vi "PIM Set Plot Colors.vi"(5 "PEAK IM":refnum<vi>, 7 "IM Plot":refnum<vi>, 8 "IM Order (0)":u8, 9 "IM In Band? (F, F, F, F)":bool[](array[boolean]), 10 "Markers Visible?":bool, 11 "DisplayMode":T1 items=["Spectral", "Strip Chart", "Swept Frequency"]) -> (2 "Mrkr Text Colors":u32[](array[numeric]), 3 "Marker Colors":u32[](array[numeric]))   [LabVIEW 2011]
uses:
  PIM Display Mode.ctl
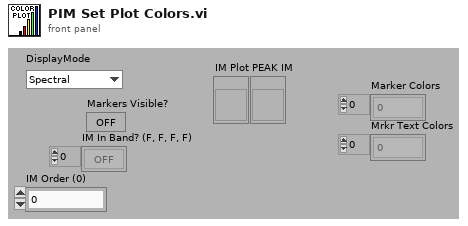
[diagram p1: front panel]
types:
  T1 = typedef "PIM Display Mode.ctl" = u16
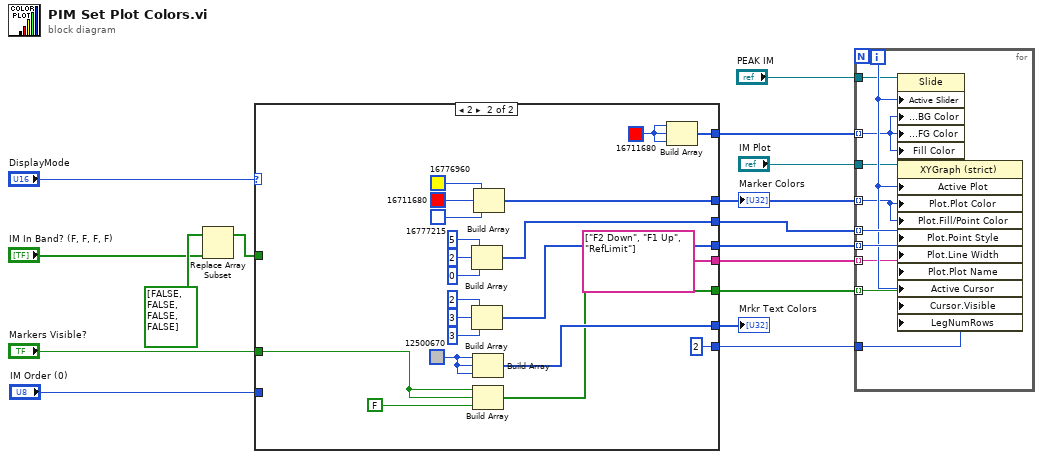
[diagram p0: block diagram]
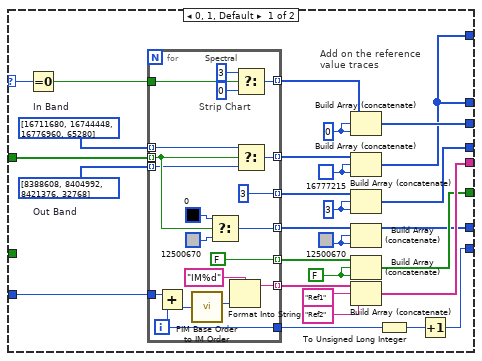
[diagram p2: hidden frame]
diagram:
  n1 = Replace Array Subset(array=bool[] [FALSE, FALSE, FALSE, FALSE], new element="IM In Band? (F, F, F, F)") -> (w1:bool[])  [unwired: 1 in]
  n2 = case shown="2" "DisplayMode" {
    selector: "DisplayMode" -> [w18 _]
    tunnel: [w36 w81] -> w15
    tunnel: [w20 w79] -> w9
    tunnel: w1 -> [w38 _]
    tunnel: [w40 w72] -> w14
    tunnel: [w19 w71] -> w13
    tunnel: "Markers Visible?" -> [_ w69]
    tunnel: [w21 w68] -> w12
    tunnel: [w36 w66] -> w7
    tunnel: [w31 string[] ["F2 Down", "F1 Up", "RefLimit"]] -> w6
    tunnel: "IM Order (0)" -> [w35 _]
    tunnel: [w28 u32 2 ("Plot.Point Style")] -> w4
    frame 0, 1, Default {
      w22 = FALSE
      w24 = u32 12500670
      w26 = u8 3 ("Plot.Point Style")
      w41 = u8 0 ("Plot.Point Style")
      w43 = u32[] [16711680, 16744448, 16776960, 65280]  # In Band
      w44 = u32[] [8388608, 8404992, 8421376, 32768]  # Out Band
      w37 = u32 16777215
      # "Add on the reference\nvalue traces"
      n3 = Equal To 0?(x=w18) -> (x = 0?=w17:bool)
      n4 = for {
        tunnel: w38 -> [w60] mode=indexing
        tunnel: w43 -> [w53] mode=indexing
        tunnel: w44 -> [w52] mode=indexing
        tunnel: [w63] -> w42 mode=indexing
        tunnel: [w59] -> w25 mode=indexing
        tunnel: [FALSE] -> w23 mode=indexing
        tunnel: [u8 3 ("Plot.Point Style")] -> w27 mode=indexing
        tunnel: [w54] -> w39 mode=indexing
        tunnel: w35 -> [w49]
        tunnel: [w47] -> w34 mode=indexing
        tunnel: [w46] -> w30
        tunnel: w17 -> [w45]
        i -> [w46]
        # "Strip Chart"
        # "Spectral"
        n5 = Add(x=w49, y=w46) -> (x+y=w48:i32)
        n6 = call "PIM Base Order to IM Order.vi"("Base Order (0)"=w48) -> ("IM Order"=w50:u8)  [unwired: 5 out]
        n7 = Select(t=u32 0, s=w60, f=u32 12500670) -> (s? t:f=w59:u32)
        n8 = Format Into String(format string="IM%d", w50) -> (resulting string=w47:string)  [unwired: 2 in, 1 out]
        n9 = Select(t=u8 3 ("Plot.Point Style"), s=w45, f=u8 0 ("Plot.Point Style")) -> (s? t:f=w54:u8)
        n10 = Select(t=w53, s=w60, f=w52) -> (s? t:f=w63:u32)
      }
      n11 = Build Array (concatenate)(w39, w41, w41) -> (w40:u8[])
      n12 = Build Array (concatenate)(w42, w37, w37) -> (w36:u32[])
      n13 = Build Array (concatenate)(w27, w26, w26) -> (w19:u8[])
      n14 = Build Array (concatenate)(w25, w24, w24) -> (w20:u32[])
      n15 = Build Array (concatenate)(w23, w22, w22) -> (w21:bool[])
      n16 = Build Array (concatenate)(w34, "Ref1" ("format string"), "Ref2" ("format string")) -> (w31:string[])
      n17 = To Unsigned Long Integer(number=w30) -> (unsigned 32bit integer=w29:u32)
      n18 = Increment(x=w29) -> (x+1=w28:u32)
    }
    frame 2 {
      w67 = u32 16711680
      w80 = u32 12500670
      n19 = Build Array(u8 5 ("Plot.Point Style"), u8 2 ("Plot.Point Style"), u8 0 ("Plot.Point Style")) -> (w72:u8[])
      n20 = Build Array(u8 2 ("Plot.Point Style"), u8 3 ("Plot.Point Style"), u8 3 ("Plot.Point Style")) -> (w71:u8[])
      n21 = Build Array(w80, w80, w80) -> (w79:u32[])
      n22 = Build Array(w69, w69, FALSE) -> (w68:bool[])
      n23 = Build Array(u32 16776960, u32 16711680, u32 16777215) -> (w81:u32[])
      n24 = Build Array(w67, w67, w67) -> (w66:u32[])
    }
  }
  "Mrkr Text Colors" <- w9
  "Marker Colors" <- w15
  n25 = for {
    tunnel: w15 -> [w88] mode=indexing
    tunnel: w14 -> [w94] mode=indexing
    tunnel: w13 -> [w93] mode=indexing
    tunnel: w12 -> [w92] mode=indexing
    tunnel: "PEAK IM" -> [w90]
    tunnel: "IM Plot" -> [w89]
    tunnel: w7 -> [w87] mode=indexing
    tunnel: w6 -> [w86] mode=indexing
    tunnel: w4 -> [w85]
    i -> [w91]
    n26 = property on="Property Node" class="Slide"(reference=w90, "Active Slider"=w91, "Slider Colors:BG Color"=w87, "Slider Colors:FG Color"=w87, "Fill Color"=w87) -> ()  [unwired: 1 in, 2 out]
    n27 = property on="Property Node" class="XYGraph (strict)"(reference=w89, "Active Plot"=w91, "Plot.Plot Color"=w88, "Plot.Fill/Point Color"=w88, "Plot.Point Style"=w94, "Plot.Line Width"=w93, "Plot.Plot Name"=w86, "Active Cursor"=w91, "Cursor.Visible"=w92, "LegNumRows"=w85) -> ()  [unwired: 1 in, 2 out]
  }
